vi "CastImage.vi"() -> ()   [LabVIEW 2018]
doc: "Use this template to build a VI to use as a subVI."
uses:
  <vilib>/vision/NI_Vision_Development_Module.lvlib
panel:
  out "L":T1(plugin-control)
  out "S":T1(plugin-control)
  out "H":T1(plugin-control)
  out "Src":T1(plugin-control)
  # ":: MVi Framework V1.0 ::\nAuthor:Gaoke Yang\nEmail: gaoke.yang@yahoo.com\nWeb: www.mvicontrol.com\nCopyright (C) 2015, MVI Technologies All Rights Reserved"
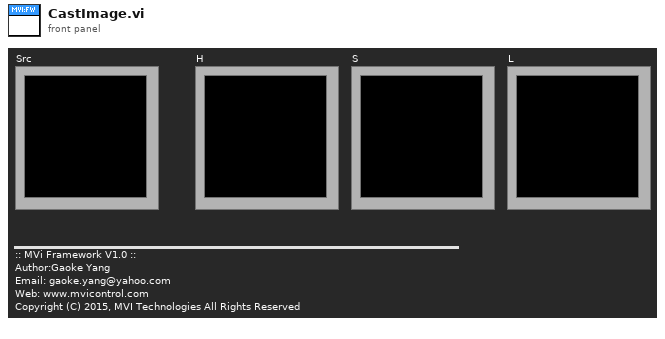
[diagram p1: front panel]
types:
  T1 = typedef "IMAQ Image.ctl" = refnum<image>
  T2 = typedef "Image Type" = u32
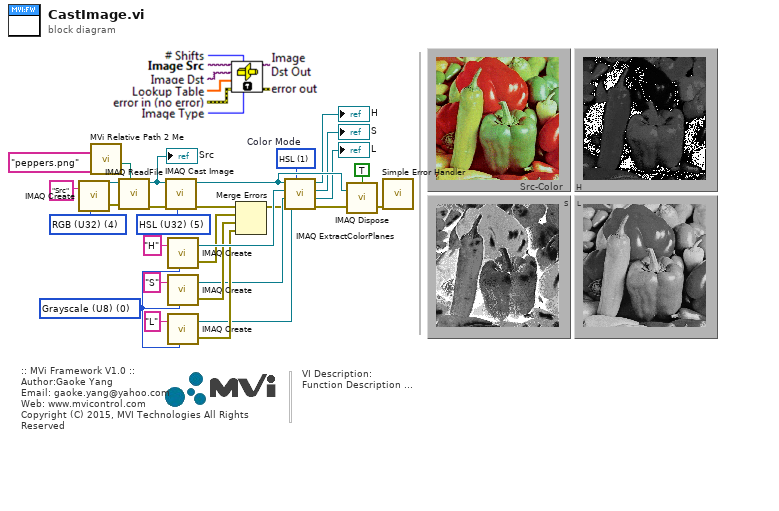
[diagram p0: block diagram]
diagram:
  w12 = T2 0 items=["Grayscale (U8)", "Grayscale (I16)", "Grayscale (SGL)", "Complex (CSG)", "RGB (U32)", "HSL (U32)", "RGB (U64)", "Grayscale (U16)"] ("Image Type")
  w20 = u16 1 items=["RGB", "HSL", "HSV", "HSI"]  # Color Mode
  w21 = T2 4 items=["Grayscale (U8)", "Grayscale (I16)", "Grayscale (SGL)", "Complex (CSG)", "RGB (U32)", "HSL (U32)", "RGB (U64)", "Grayscale (U16)"] ("Image Type")
  w22 = T2 5 items=["Grayscale (U8)", "Grayscale (I16)", "Grayscale (SGL)", "Complex (CSG)", "RGB (U32)", "HSL (U32)", "RGB (U64)", "Grayscale (U16)"] ("Image Type")
  # "L"
  # "S"
  # "H"
  # "Src-Color"
  # "VI Description:\nFunction Description ..."
  # ":: MVi Framework V1.0 ::\nAuthor:Gaoke Yang\nEmail: gaoke.yang@yahoo.com\nWeb: www.mvicontrol.com\nCopyright (C) 2015, MVI Technologies All Rights Reserved"
  n1 = call "IMAQ Create"("Image Name"="Src" ("name or relative path"), "Image Type"=w21) -> ("New Image"=w25:T1, "error out"=w24:errorcluster)  [unwired: 2 in, 1 out]
  n2 = call "MVi Relative Path 2 Me.vi"("Relative Path"="peppers.png" ("name or relative path")) -> ("Appended Dir"=w1:path)  [unwired: 5 in, 1 out]
  n3 = call "IMAQ ReadFile"("File Path"=w1, "error in (no error)"=w24, "Image"=w25) -> ("error out"=w23:errorcluster, "Image Out"=w16:T1)  [unwired: 4 in, 3 out]
  "Src" <- w16
  n4 = call "IMAQ Cast Image"("Image Type"=w22, "error in (no error)"=w23, "Image Src"=w16) -> ("error out"=w8:errorcluster, "Image Dst Out"=w29:T1)  [unwired: 7 in]
  n5 = call "IMAQ Create"("Image Name"="H" ("name or relative path"), "Image Type"=w12) -> ("New Image"=w17:T1, "error out"=w11:errorcluster)  [unwired: 2 in, 1 out]
  n6 = call "IMAQ Create"("Image Name"="S" ("name or relative path"), "Image Type"=w12) -> ("New Image"=w7:T1, "error out"=w10:errorcluster)  [unwired: 2 in, 1 out]
  n7 = call "IMAQ Create"("Image Name"="L" ("name or relative path"), "Image Type"=w12) -> ("New Image"=w6:T1, "error out"=w9:errorcluster)  [unwired: 2 in, 1 out]
  n8 = Merge Errors(w8, w11, w10, w9) -> (w5:errorcluster)
  n9 = call "IMAQ ExtractColorPlanes"("Blue or Luma or Val or Inten Plane"=w6, "Color Mode"=w20, "error in (no error)"=w5, "Green or Sat Plane"=w7, "Red or Hue Plane"=w17, "Image Src"=w29) -> ("error out"=w19:errorcluster, "Blue or Luma or Val or Inten Plane out"=→"L":T1, "Green or Sat Plane out"=→"S":T1, "Red or Hue Plane out"=→"H":T1)  [unwired: 2 in]
  n10 = call "IMAQ Dispose"("All Images? (No)"=TRUE, "Image"=w29, "error in (no error)"=w19) -> ("error out"=w26:errorcluster)  [unwired: 3 out]
  n11 = call <vilib>:"Simple Error Handler.vi"("error in (no error)"=w26) -> ()  [unwired: 1 in, 8 out]
